vi "Global Variables.vi"() -> ()   [LabVIEW 2018]
panel:
  in  "Repository path":path=path "C:/Users/aspitarl/Git/MHDLab"
  in  "Data folder":path=path "C:/Labview Test Data"
  in  "Delta T":dbl=1.0
  in  "F-m'":dbl=0.0006116654518407403
  in  "Global File Information":T1={"Project"=0, "SubFolder"="Temp Dependence", "Filename (Meas. Description)"="400C", "Measurement index"=0} {"Project" items=["Proj_Vaportubes", "Proj_H2DT"]}
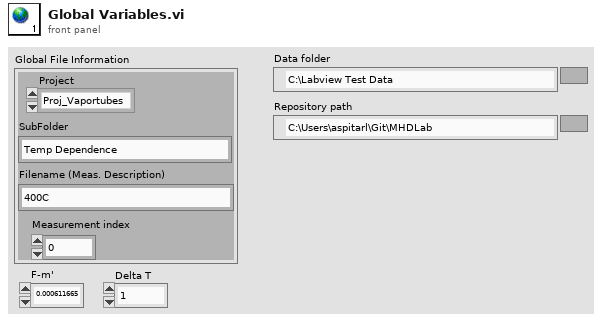
[diagram p1: front panel]
types:
  T1 = cluster{"Project":u16, "SubFolder":string, "Filename (Meas. Description)":string, "Measurement index":i32}
diagram:
